vi "Format File URL.vi"(0 "file name":string, 5 "file dir":path, 7 "base dir":path, 11 "Use HTML Space Formating (%20)":bool) -> (4 "image URL string":string)   [LabVIEW 2019, in "MD Generator.lvlib"]
uses:
  MD Generator.lvlib
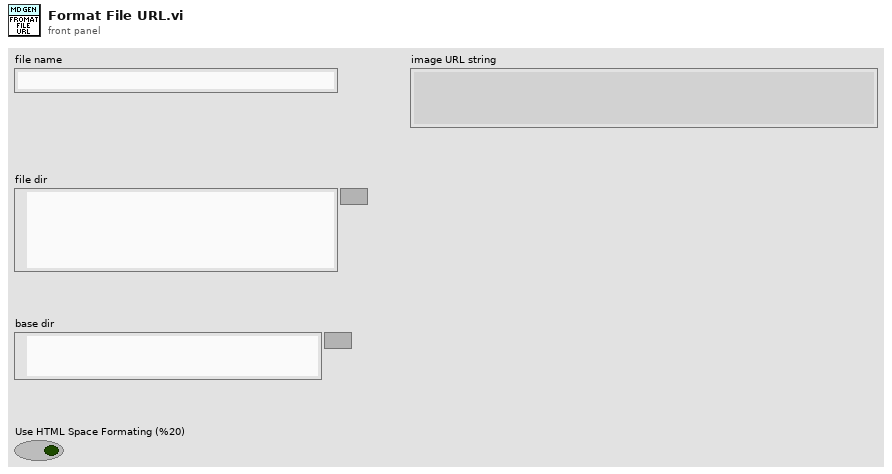
[diagram p1: front panel]
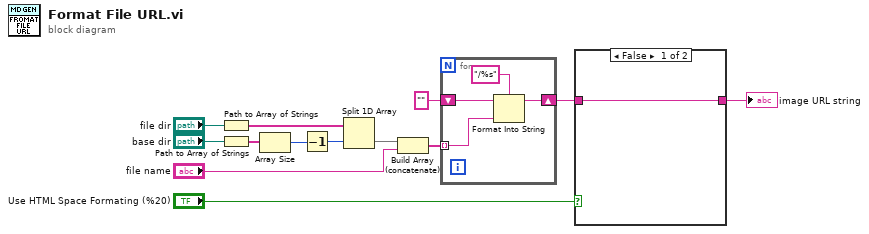
[diagram p0: block diagram]
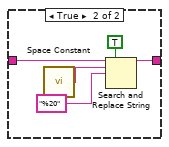
[diagram p2: hidden frame]
diagram:
  n1 = Path to Array of Strings(0:"file dir") -> (2:w8:string[])  [unwired: 1 out]
  n2 = Path to Array of Strings(0:"base dir") -> (2:w9:string[])  [unwired: 1 out]
  n3 = Array Size(array=w9) -> (size(s)=w10:i32)
  n4 = Decrement(x=w10) -> (x-1=w2:i32)
  n5 = Split 1D Array(array=w8, index=w2) -> (second subarray=w7:string[])  [unwired: 1 out]
  n6 = Build Array (concatenate)(w7, "file name") -> (w5:string[])
  n7 = for {
    shift-right: [w16] -> w4
    shift-left: "" -> [w17]
    tunnel: w5 -> [w14] mode=indexing
    n8 = Format Into String(format string="/%s", initial string=w17, w14) -> (resulting string=w16:string)  [unwired: 1 in, 1 out]
  }
  n9 = case shown="False" "Use HTML Space Formating (%20)" {
    tunnel: w4 -> [w18 w23]
    tunnel: [w18 w20] -> w3
    frame False {
    }
    frame True {
      n10 = call <vilib>:"Space Constant.vi"() -> ("String"=w22:string)
      n11 = Search and Replace String(replace all?=TRUE ("replace all? (F)"), input string=w23, search string=w22, replace string="%20" ("replace string (\"\")")) -> (result string=w20:string)  [unwired: 4 in, 3 out]
    }
  }
  "image URL string" <- w3
